vi "exercicios7_structures.vi"() -> ()   [LabVIEW 2018]
panel:
  in  "stop":bool
  out "Waveform Graph 2":dbl[](graph)
  in  "Slide":dbl(slide) scale=0.0..1000.0
  out "Array":i32[](array[numeric])
  out "Waveform Graph":dbl[](graph)
  out "output variable":dbl
  out "Color":u32(colorbox)
  # "Exercício 3"
  # "Exercício 4"
  # "Exercício 1"
  # "Exercício 2"
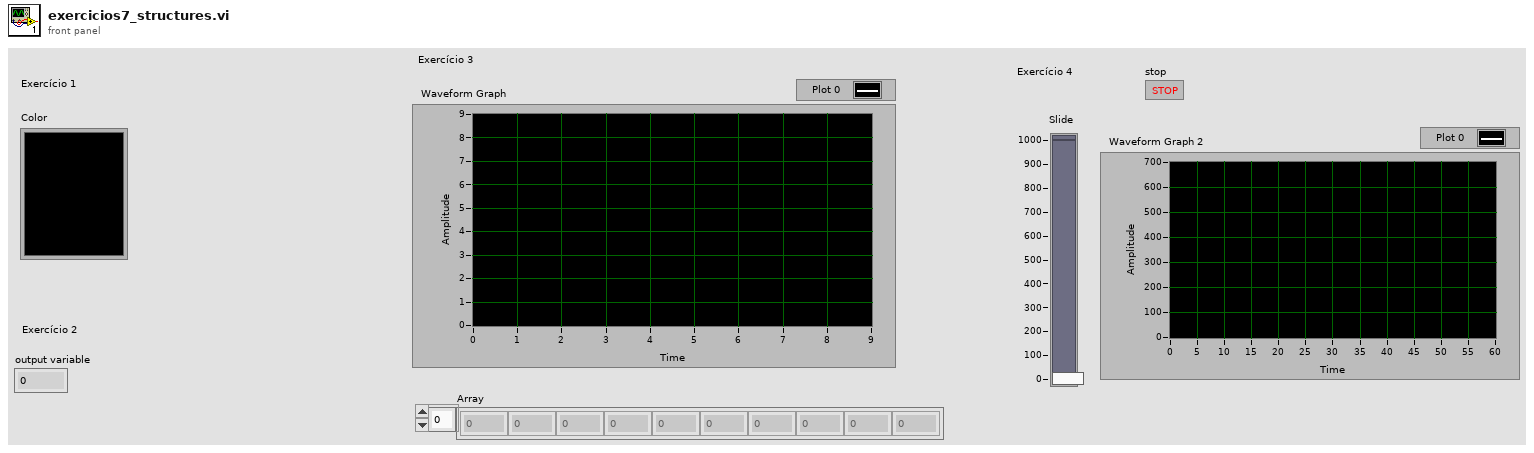
[diagram p1: front panel]
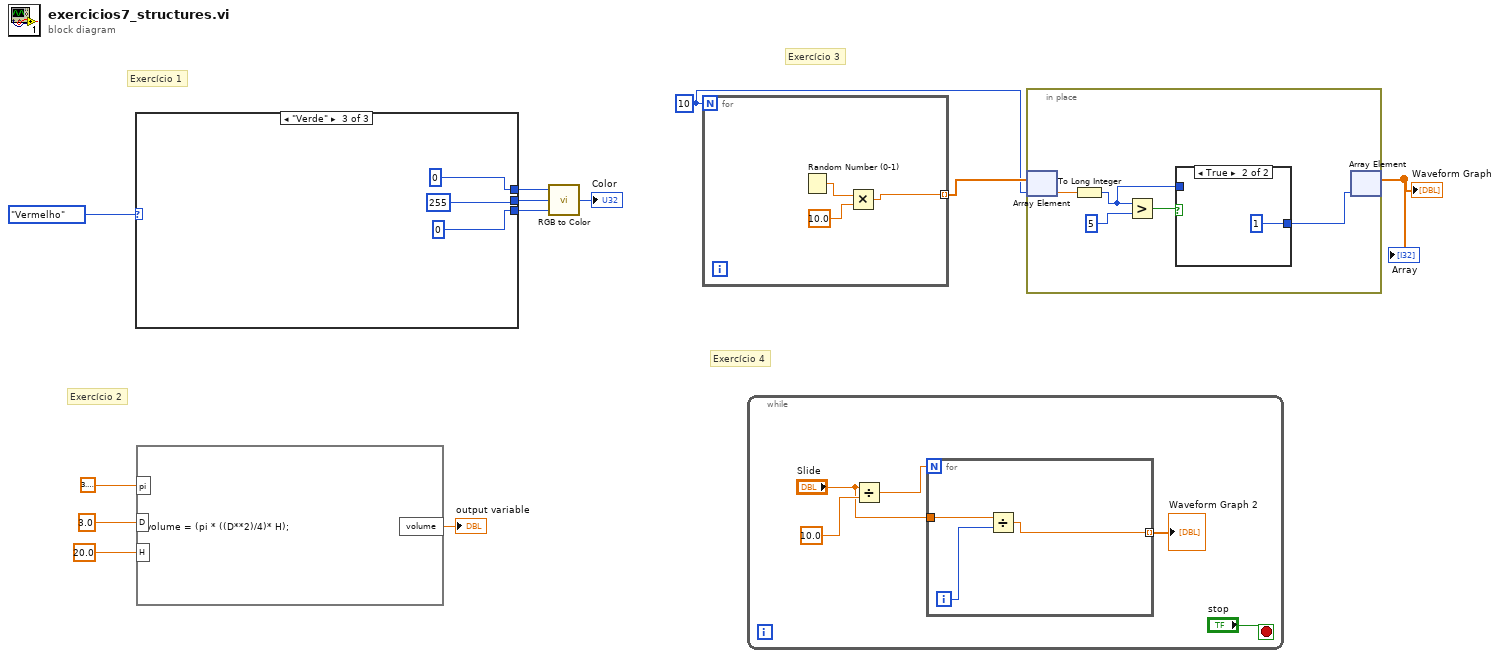
[diagram p0: block diagram]
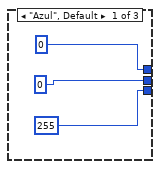
[diagram p3: hidden frame]
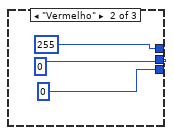
[diagram p4: hidden frame]
diagram:
  w1 = 10
  # "Exercício 4"
  # "Exercício 3"
  # "Exercício 2"
  # "Exercício 1"
  n1 = case shown="\"Verde\"" enum16{"Azul", "Vermelho", "Verde"}."Vermelho" {
    tunnel: [0 255 0] -> w11
    tunnel: [0 0 255] -> w10
    tunnel: [255 0 0] -> w9
    frame "Azul", Default {
    }
    frame "Vermelho" {
    }
    frame "Verde" {
    }
  }
  n2 = formula code="volume = (pi * ((D**2)/4)* H);"("pi"=3.141592653589793, "D"=3.0 ("input variable"), "H"=20.0 ("input variable")) -> ("volume"=→"output variable":dbl)
  n3 = call <vilib>:"RGB to Color.vi"("B"=w9, "G"=w10, "R"=w11) -> ("Color"=→"Color":u32)
  n4 = for {
    N: w1 -> [_]
    tunnel: [w22] -> w3 mode=indexing
    n5 = Random Number (0-1)() -> (number: 0 to 1=w24:dbl)
    n6 = Multiply(x=w24, y=10.0) -> (x*y=w22:dbl)
  }
  n7 = while {
    stop <- "stop" stop-if-true
    n8 = Divide(x="Slide", y=10.0) -> (x/y=w28:dbl)
    n9 = for {
      N: w28 -> [_]
      tunnel: "Slide" -> [w32]
      tunnel: [w30] -> w26 mode=indexing
      i -> [w31]
      n10 = Divide(x=w32, y=w31) -> (x/y=w30:dbl)
    }
    "Waveform Graph 2" <- w26
  }
  n11 = in-place {
    n12 = in-place-array #1(w3, w1) -> (w37:dbl)
    n13 = To Long Integer(number=w37) -> (32bit integer=w34:i32)
    n14 = Greater?(x=w34, y=5) -> (0:w33:bool)
    n15 = case shown="True" w33 {
      tunnel: [w38 1] -> w35
      tunnel: w34 -> [w38 _]
      frame False {
      }
      frame True {
      }
    }
    n16 = in-place-array #1(w35) -> (→"Waveform Graph" →"Array":dbl[])  [unwired: 1 out]
  }
